vi "mupExpr multiExpr multiVar example2.vi"() -> ()   [LabVIEW 2015]
uses:
  mupExpr/mupExpr.lvclass
  mupExpr/mupExpr.lvclass/mupExpr.ctl
  mupExpr/Eval_MultiVar_SglRes.vi
  mupExpr/SetVarVal.vi
  mupLib/mupEval.vi
  mupLib/mupSetVarValue.vi
  mupLib/mupCheckError.vi
  mupLib/mupLibPath.vi
  <vilib>/Utility/error.llb/Error Cluster From Error Code.vi
panel:
  out "error out":errorcluster
  out "varValues out":dbl[](array[numeric]) format="%#_13g"
  out "Variable Names":string[](array[string])
  in  "Expression":string="y = sin(w*x+c),\nz = a*x^2+b*x+c,\nr = a*x+b"
  in  "Variable Values":dbl[](array[numeric])=[1.0, 2.0, 3.0, 3.141592654, 1.0, 0.0, 0.0, 0.0] format="%#_13g"
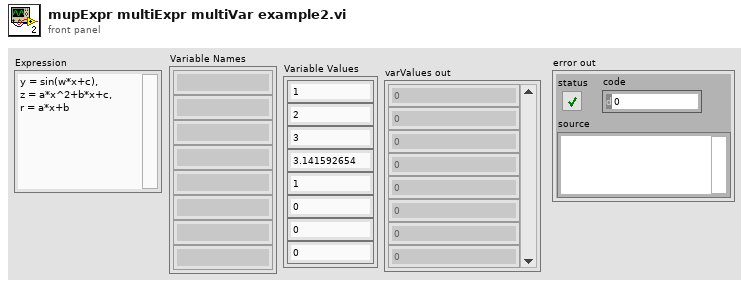
[diagram p1: front panel]
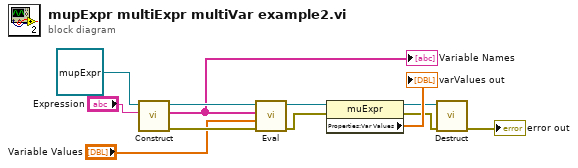
[diagram p0: block diagram]
diagram:
  n1 = call-dynamic "Construct.vi"("Expression"="Expression", "muExpr in"=refnum<class "mupExpr.lvclass"> refnum) -> ("error out"=w12:errorcluster, "Variable Names"=w7:string[], "mupExpr out"=w11:refnum<class "mupExpr.lvclass">)  [unwired: 6 in, 1 out]
  "Variable Names" <- w7
  n2 = call-poly "Eval.vi"("error in (no error)"=w12, "varValues"="Variable Values", "varNames"=w7, "muExpr in"=w11) -> ("error out"=w5:errorcluster, "muExpr out"=w6:refnum<class "mupExpr.lvclass">)  [unwired: 5 in, 1 out]
  n3 = property class="muExpr"(reference=w6, error in=w5) -> (reference out=w3:refnum<class "mupExpr.lvclass">, error out=w2:errorcluster, "Properties:Var Values"=→"varValues out":dbl[])
  n4 = call-dynamic "Destruct.vi"("error in (no error)"=w2, "muExpr in"=w3) -> ("error out"=→"error out":errorcluster)  [unwired: 9 in]
